vi "Sub_VI_analiza_kolorow.vi"(11 "u":dbl) -> (3 "Cluster":T1)   [LabVIEW 2020]
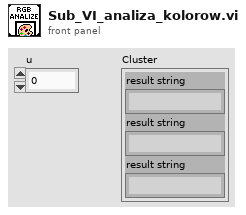
[diagram p1: front panel]
types:
  T1 = cluster{"result string":string, "result string":string, "result string":string}
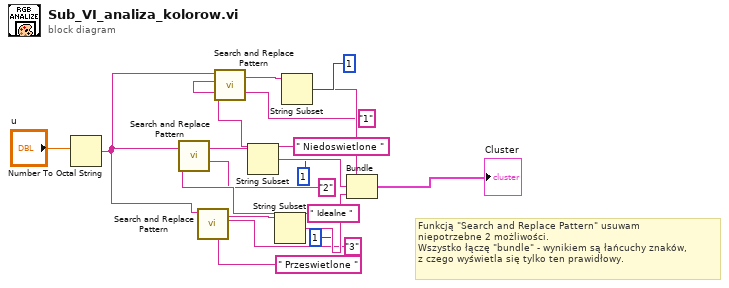
[diagram p0: block diagram]
diagram:
  # "Funkcją \"Search and Replace Pattern\" usuwam\nniepotrzebne 2 możliwości.\nWszystko łączę \"bundle\" - wynikiem są łańcuchy znaków,\nz czego wyświetla się tylko ten prawidłowy."
  n1 = Number To Octal String(2:"u") -> (0:w7:string)  [unwired: 1 in]
  n2 = call <vilib>:"Search and Replace Pattern.vi"("string"=w7, "regular expression (\"\")"="2" ("regular expression (\"\")"), "replace string (\"\")"=" Idealne " ("replace string (\"\")")) -> ("result string"=w10:string)  [unwired: 2 in, 1 out]
  n3 = call <vilib>:"Search and Replace Pattern.vi"("string"=w7, "regular expression (\"\")"="3" ("regular expression (\"\")"), "replace string (\"\")"=" Przeswietlone " ("replace string (\"\")")) -> ("result string"=w13:string)  [unwired: 2 in, 1 out]
  n4 = call <vilib>:"Search and Replace Pattern.vi"("string"=w7, "regular expression (\"\")"="1" ("regular expression (\"\")"), "replace string (\"\")"=" Niedoswietlone " ("replace string (\"\")")) -> ("result string"=w11:string)  [unwired: 2 in, 1 out]
  n5 = String Subset(string=w10, offset (0)=1) -> (substring=w14:string)  [unwired: 1 in]
  n6 = String Subset(string=w13, offset (0)=1) -> (substring=w15:string)  [unwired: 1 in]
  n7 = String Subset(string=w11, offset (0)=1) -> (substring=w12:string)  [unwired: 1 in]
  n8 = Bundle("result string"=w12, "result string"=w14, "result string"=w15) -> (→"Cluster":T1)  [unwired: 1 in]
